vi "Fetch And Remove.vi"(8 "error in (no error)":errorcluster {"code" format="%.0x"}, 9 "ValBufferSize":i32=2048, 10 "Count":i32 format="%.0g", 11 "instrument handle":refnum<k15>) -> (0 "error out":errorcluster {"code" format="%.0x"}, 2 "Val":string, 3 "instrument handle out":refnum<k15>)   [LabVIEW 2020, in "Keysight DAQ970.lvlib"]
doc: "Returns and clears the specified number of scan data readings from non-volatile memory starting with the oldest reading. This allows you to continue a scan without losing data stored in memory (if memory becomes full, new readings overwrite oldest readings)."
uses:
  Keysight DAQ970.lvlib
  KtDAQ970.dll
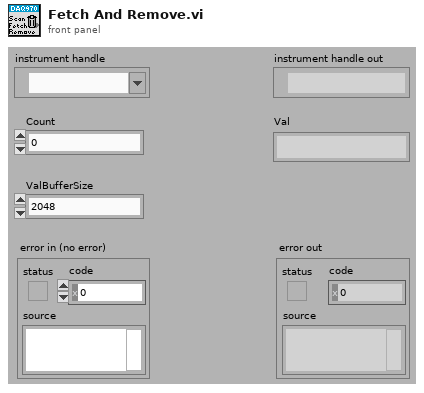
[diagram p1: front panel]
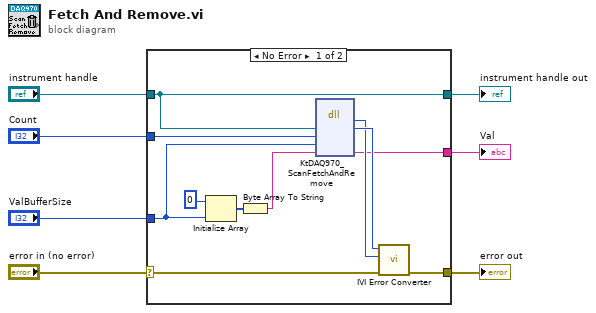
[diagram p0: block diagram]
diagram:
  n1 = case shown="No Error" "error in (no error)" {
    selector: "error in (no error)" -> [w16 w20]
    tunnel: [w15 w20] -> w7
    tunnel: "instrument handle" -> [w9 w19]
    tunnel: "Count" -> [w14 _]
    tunnel: "ValBufferSize" -> [w8 _]
    tunnel: [w10 _] -> w2
    tunnel: [w9 w19] -> w1
    frame No Error {
      n2 = Initialize Array(u8 0 ("element"), w8) -> (w12:u8[])
      n3 = Byte Array To String(unsigned byte array=w12) -> (string=w13:string)
      n4 = dll-call lib="KtDAQ970**.dll" fn="KtDAQ970_ScanFetchAndRemove"("Vi"=w9, "Count"=w14, "ValBufferSize"=w8, "Val"=w13) -> (w17:i32, "Vi"=w18:u32, "Val"=w10:string)  [unwired: 5 in, 2 out]
      n5 = call "IVI Error Converter.vi"("error in (no error)"=w16, "IVI error code (0)"=w17, "instrument handle"=w18) -> ("error out"=w15:errorcluster)  [unwired: 7 in, 1 out]
    }
    frame Error {
    }
  }
  "error out" <- w7
  "instrument handle out" <- w1
  "Val" <- w2
